vi "T5.vi"() -> ()   [LabVIEW 2020]
panel:
  out "B":dbl
  in  "A":dbl
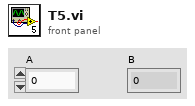
[diagram p1: front panel]
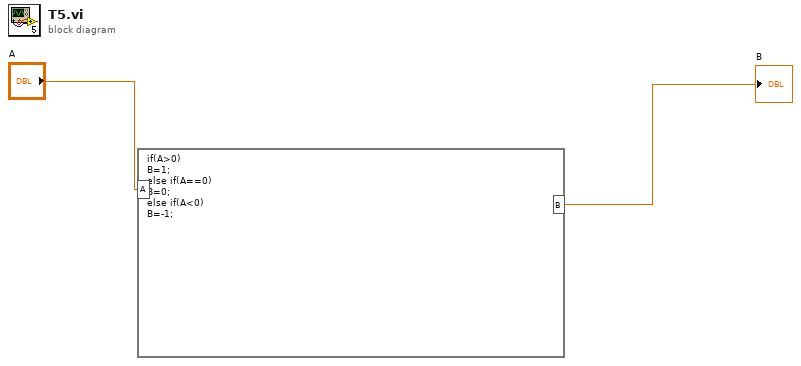
[diagram p0: block diagram]
diagram:
  n1 = formula code="if(A>0) \nB=1;\nelse if(A==0)\nB=0;\nelse if(A<0)\nB=-1;"("A"="A") -> ("B"=→"B":dbl)
